vi "tmp_toml_sections.vi"(4 "vi":refnum<vi>, 8 "error in (no error)":errorcluster, 11 "path in":path) -> (0 "error out":errorcluster, 1 "sections":string[](array[string]), 2 "file exists":bool, 3 "path out":path)   [LabVIEW 2017]
uses:
  <vilib>/Utility/error.llb/Clear Errors.vi
  <vilib>/Utility/file.llb/Application Directory.vi
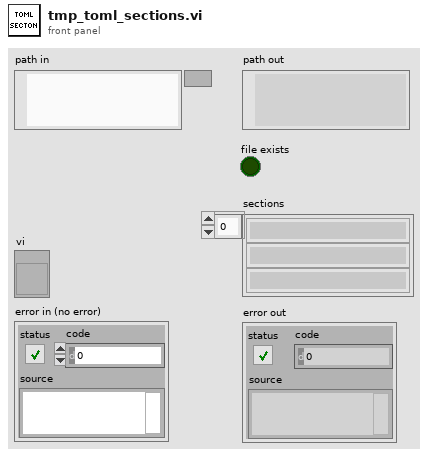
[diagram p1: front panel]
types:
  T1 = enum16{"open", "replace", "create", "open or create", "replace or create", "replace or create with confirmation"}
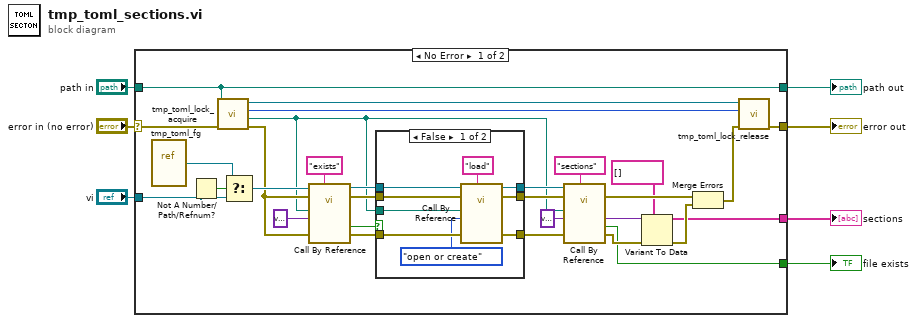
[diagram p0: block diagram]
diagram:
  n1 = case shown="No Error" "error in (no error)" {
    selector: "error in (no error)" -> [w35 w50]
    tunnel: [w32 w50] -> w6
    tunnel: "vi" -> [w29 _]
    tunnel: "path in" -> [w27 w51]
    tunnel: [w27 w51] -> w3
    tunnel: [w25 _] -> w2
    tunnel: [w16 _] -> w1
    frame No Error {
      n2 = vi-ref "tmp_toml_fg.vi"() -> (w28:refnum<vi>)
      n3 = Not A Number/Path/Refnum?(number/path/refnum=w29) -> (NaN/Path/Refnum?=w30:bool)
      n4 = call "tmp_toml_lock_acquire.vi"("error in (no error)"=w35, "path in"=w27) -> ("error out"=w22:errorcluster, "resolved path"=w8:path, "cnt"=w36:u8, "lock"=w37:refnum<queue>)  [unwired: 6 in]
      n5 = Select(t=w28, s=w30, f=w29) -> (s? t:f=w23:refnum<vi>)
      n6 = call-by-ref "?"(reference=w23, error in=w22, "cmd"="exists", 8:"error in (no error)"=w22, "data in"=variant, "path in"=w8) -> (reference out=w15:refnum<vi>, error out=w14:errorcluster, 0:"error out"=w13:errorcluster, "return"=w9:bool)  [unwired: 4 in, 2 out]
      n7 = case shown="False" w9 {
        tunnel: w15 -> [w46 w49]
        tunnel: w14 -> [w45 w48]
        tunnel: w13 -> [w44 w47]
        tunnel: [w43 w47] -> w12
        tunnel: [w42 w48] -> w11
        tunnel: [w41 w49] -> w10
        tunnel: w8 -> [w39 _]
        frame False {
          n8 = call-by-ref "?"(reference=w46, error in=w45, "cmd"="load", 8:"error in (no error)"=w44, "data in"=T1."open or create" ("operation (open or create)"), "path in"=w39) -> (reference out=w41:refnum<vi>, error out=w42:errorcluster, 0:"error out"=w43:errorcluster)  [unwired: 4 in, 3 out]
        }
        frame True {
        }
      }
      n9 = call-by-ref "?"(reference=w10, error in=w11, "cmd"="sections", 8:"error in (no error)"=w12, "data in"=variant, "path in"=w8) -> (error out=w34:errorcluster, 0:"error out"=w26:errorcluster, "return"=w25:bool, "data out"=w18:variant)  [unwired: 4 in, 2 out]
      n10 = Variant To Data(error in=w26, type=string[] [], Variant=w18) -> (data=w16:string[], error out=w19:errorcluster)
      n11 = Merge Errors(w34, w19) -> (w33:errorcluster)
      n12 = call "tmp_toml_lock_release.vi"("error in (no error)"=w33, "cnt"=w36, "lock"=w37) -> ("error out"=w32:errorcluster)  [unwired: 8 in]
    }
    frame Error {
    }
  }
  "error out" <- w6
  "path out" <- w3
  "file exists" <- w2
  "sections" <- w1
